vi "Read Config.vi"(8 "error in (no error)":errorcluster, 9 "Re-Init?":bool, 10 "ICM File In":path, 11 "Query in":refnum<class "Query.lvclass">) -> (0 "error out":errorcluster, 3 "Query out":refnum<class "Query.lvclass">)   [LabVIEW 2018, in "Query.lvclass"]
doc: "Query.lvclass:Read Config.vi\n\nThis is the template for the Read Config VI for the Query class.\n\nInstrument Communication Module Version 1.0\nSeptember, 2017 Original Code Consulting David Thomson\n www.originalcode.com"
uses:
  Query.lvclass
  Query.lvclass/Query.ctl
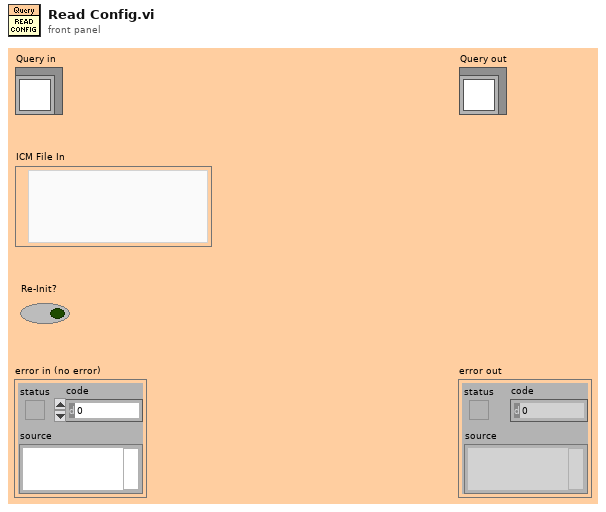
[diagram p1: front panel]
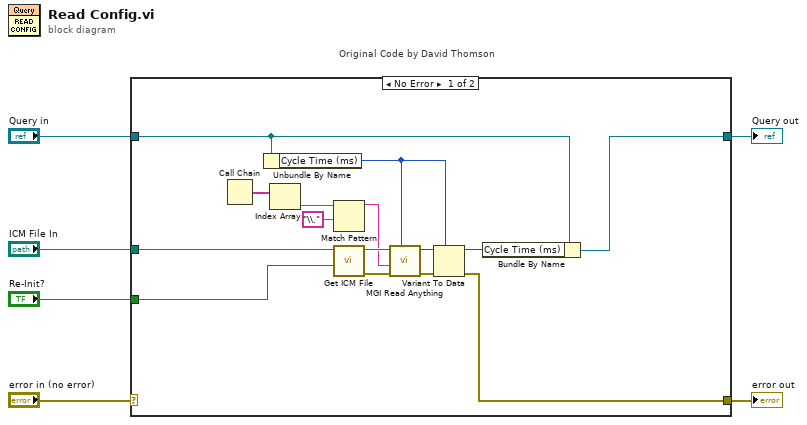
[diagram p0: block diagram]
diagram:
  n1 = case "Original Code by David Thomson" shown="No Error" "error in (no error)" {
    selector: "error in (no error)" -> [_ w23]
    tunnel: [w9 w23] -> w5
    tunnel: [w10 w22] -> w3
    tunnel: "Query in" -> [w11 w22]
    tunnel: "ICM File In" -> [w8 _]
    tunnel: "Re-Init?" -> [w7 _]
    frame No Error {
      n2 = Call Chain() -> (call chain=w18:string[])
      n3 = Unbundle By Name(w11) -> ("Cycle Time (ms)"=w12:u32)
      n4 = Index Array(array=w18) -> (element=w19:string)  [unwired: 1 in]
      n5 = Match Pattern(string=w19, regular expression="\\.") -> (before substring=w16:string)  [unwired: 1 in, 3 out]
      n6 = call "Get ICM File.vi"("Re-Init?"=w7, "ICM File In"=w8) -> ("error out"=w20:errorcluster, "ICM File"=w21:path)  [unwired: 8 in]
      n7 = call "MGI Read Anything.vi"("Type of Anything"=w12, "Error In"=w20, "Section Name (Name of \"Type of Anything\")"=w16, "Path (dialog)"=w21) -> ("Error Out"=w14:errorcluster, "Anything"=w15:variant)  [unwired: 4 in, 2 out]
      n8 = Variant To Data(error in=w14, type=w12, Variant=w15) -> (data=w13:u32, error out=w9:errorcluster)
      n9 = Bundle By Name(cluster=w11, "Cycle Time (ms)"=w13) -> (w10:refnum<class "Query.lvclass">)
    }
    frame Error {
    }
  }
  "error out" <- w5
  "Query out" <- w3
